vi "Read.vi"(8 "error in":errorcluster, 11 "VISA resource name":refnum<visa-resource-name>) -> (0 "error out":errorcluster, 1 "Length":u32, 2 "Message":string, 3 "VISA resource name out":refnum<visa-resource-name>)   [LabVIEW 2017, in "Andeen-Hagerling 2700.lvlib"]
doc: "Read all available bytes from the selected VISA resource."
uses:
  Andeen-Hagerling 2700.lvlib
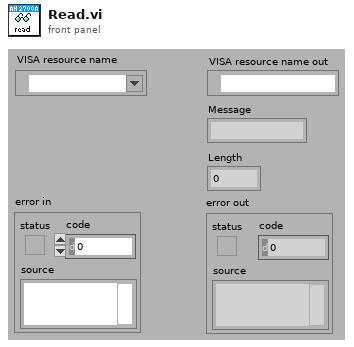
[diagram p1: front panel]
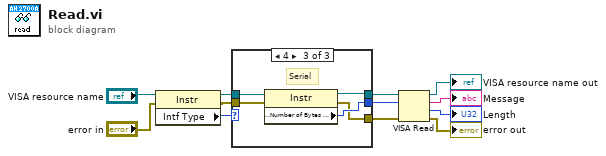
[diagram p0: block diagram]
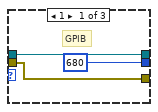
[diagram p2: hidden frame]
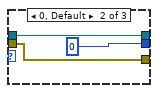
[diagram p3: hidden frame]
diagram:
  n1 = property class="Instr"(reference="VISA resource name", error in="error in") -> (reference out=w11:refnum<visa-resource-name>, error out=w5:errorcluster, "Intf Type"=w12:u16)
  n2 = case shown="4" w12 {
    tunnel: w11 -> [w14 w18 w23]
    tunnel: [w14 w18 w21] -> w10
    tunnel: [w13 w16 w20] -> w9
    tunnel: [u16 680 ("y") u32 0 ("Bytes at Port") w22] -> w8
    tunnel: w5 -> [w13 w16 w19]
    frame 1 {
      # "GPIB"
    }
    frame 0, Default {
    }
    frame 4 {
      # "Serial"
      n3 = property class="Instr"(reference=w23, error in=w19) -> (reference out=w21:refnum<visa-resource-name>, error out=w20:errorcluster, "Serial Settings:Number of Bytes at Serial Port"=w22:u32)
    }
  }
  n4 = VISA Read(VISA resource name=w10, byte count=w8, error in (no error)=w9) -> (VISA resource name out=→"VISA resource name out":refnum<visa-resource-name>, read buffer=→"Message":string, return count=→"Length":u32, error out=→"error out":errorcluster)
